vi "RPM target.vi"(6 "error constant":dbl, 7 "PWM IN":dbl, 8 "RPM MAX":u64, 9 "Voltage IN":u32, 10 "RPM IN":u64, 11 "elapsed ms":u32) -> (0 "PWM":dbl, 1 "Voltage OUT":u32, 3 "New Target RPM":u64)   [LabVIEW 2013]
panel:
  in  "RPM range":u64=250
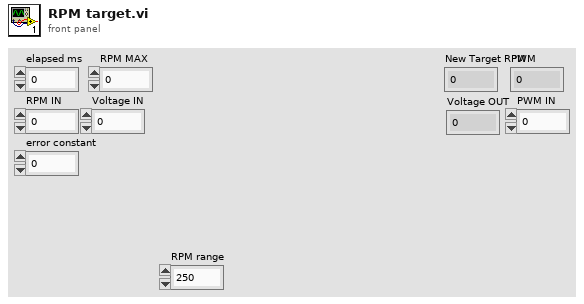
[diagram p1: front panel]
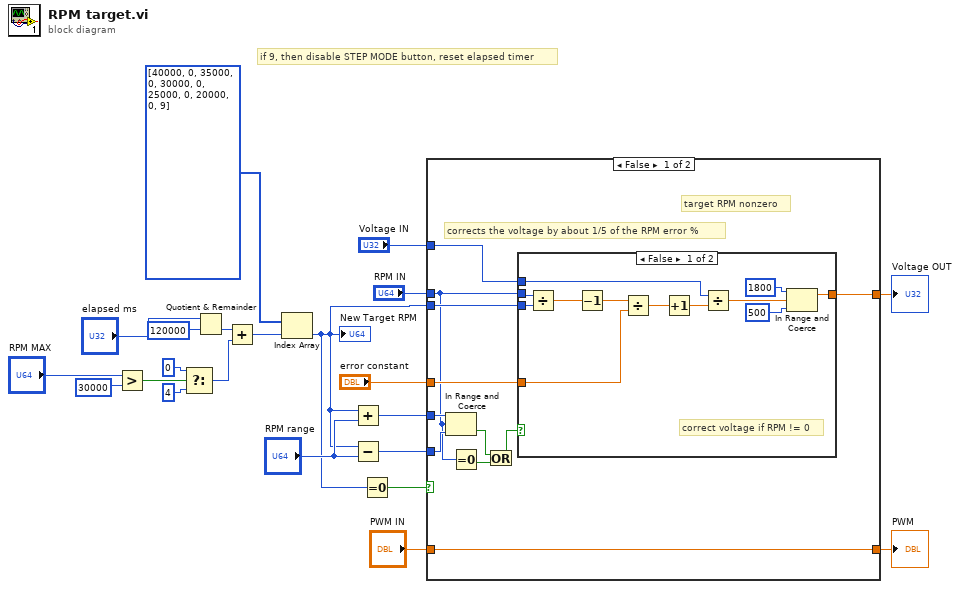
[diagram p0: block diagram]
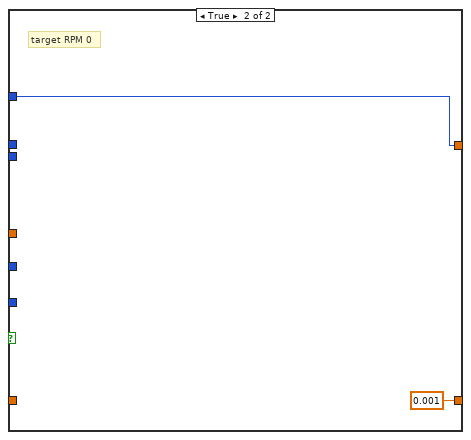
[diagram p3: hidden frame]
diagram:
  # "if 9, then disable STEP MODE button, reset elapsed timer"
  n1 = Greater?(x="RPM MAX", y=u64 30000) -> (0:w14:bool)
  n2 = Select(t=u32 0 ("y"), s=w14, f=u32 4 ("y")) -> (s? t:f=w10:u32)
  n3 = Quotient & Remainder(x="elapsed ms", y=u32 120000) -> (floor(x/y)=w6:u32)  [unwired: 1 out]
  n4 = Add(x=w6, y=w10) -> (x+y=w11:u32)
  n5 = Index Array(array=u64[] [40000, 0, 35000, 0, 30000, 0, 25000, 0, 20000, 0, 9], index=w11) -> (element=w1:u64)
  "New Target RPM" <- w1
  n6 = Add(x=w1, y="RPM range") -> (x+y=w21:u64)
  n7 = Subtract(x=w1, y="RPM range") -> (x-y=w20:u64)
  n8 = Equal To 0?(x=w1) -> (x = 0?=w2:bool)
  n9 = case shown="False" w2 {
    tunnel: w21 -> [w33 _]
    tunnel: w20 -> [w32 _]
    tunnel: [w31 w48] -> w9
    tunnel: "Voltage IN" -> [w30 w48]
    tunnel: "RPM IN" -> [w26 _]
    tunnel: "error constant" -> [w29 _]
    tunnel: w1 -> [w28 _]
    tunnel: [w27 0.001 ("f")] -> w4
    tunnel: "PWM IN" -> [w27 _]
    frame False {
      # "target RPM nonzero"
      # "corrects the voltage by about 1/5 of the RPM error %"
      n10 = In Range and Coerce(upper limit=w33, x=w26, lower limit=w32) -> (In Range?=w24:bool)  [unwired: 1 out]
      n11 = Equal To 0?(x=w26) -> (x = 0?=w25:bool)
      n12 = Or(x=w24, y=w25) -> (x .or. y?=w23:bool)
      n13 = case shown="False" w23 {
        tunnel: [w42 w46] -> w31
        tunnel: w30 -> [w43 w46]
        tunnel: w28 -> [w44 _]
        tunnel: w26 -> [w45 _]
        tunnel: w29 -> [w37 _]
        frame False {
          # "correct voltage if RPM != 0"
          n14 = Divide(x=w45, y=w44) -> (x/y=w38:dbl)
          n15 = Decrement(x=w38) -> (x-1=w35:dbl)
          n16 = Divide(x=w35, y=w37) -> (x/y=w36:dbl)
          n17 = Increment(x=w36) -> (x+1=w34:dbl)
          n18 = Divide(x=w43, y=w34) -> (x/y=w39:dbl)
          n19 = In Range and Coerce(upper limit=u32 1800 ("y"), x=w39, lower limit=u32 500 ("y")) -> (coerced(x)=w42:dbl)  [unwired: 1 out]
        }
        frame True {
          # "target acquired"
        }
      }
    }
    frame True {
      # "target RPM 0"
    }
  }
  "Voltage OUT" <- w9
  "PWM" <- w4
